vi "Example Bundler 2.vi"() -> ()   [LabVIEW 2014]
panel:
  out "ClusterIndicatorMy":cluster{string, i32, string[]}
  out "Error Out":errorcluster
  in  "Error In":errorcluster
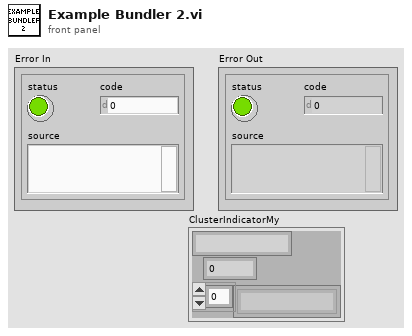
[diagram p1: front panel]
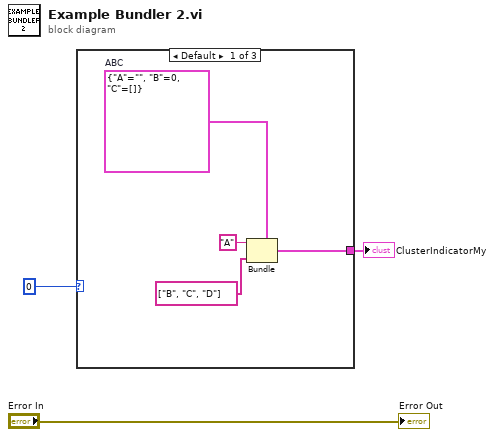
[diagram p0: block diagram]
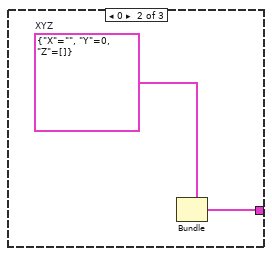
[diagram p2: hidden frame]
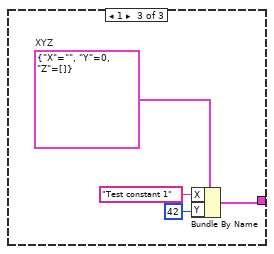
[diagram p3: hidden frame]
diagram:
  n1 = case shown="Default" 0 {
    tunnel: [w4 w8 w10] -> w1
    frame Default {
      w7 = cluster{"A":string, "B":i32, "C":string[]} {"A"="", "B"=0, "C"=[]}  # ABC
      n2 = Bundle(cluster=w7, "A"="A", "C"=string[] ["B", "C", "D"]) -> (w4:cluster{"A":string, "B":i32, "C":string[]})  [unwired: 1 in]
    }
    frame 0 {
      w9 = cluster{"X":string, "Y":i32, "Z":string[]} {"X"="", "Y"=0, "Z"=[]}  # XYZ
      n3 = Bundle(cluster=w9) -> (w8:cluster{"X":string, "Y":i32, "Z":string[]})  [unwired: 3 in]
    }
    frame 1 {
      w13 = cluster{"X":string, "Y":i32, "Z":string[]} {"X"="", "Y"=0, "Z"=[]}  # XYZ
      n4 = Bundle By Name(cluster=w13, "X"="Test constant 1", "Y"=42) -> (w10:cluster{"X":string, "Y":i32, "Z":string[]})
    }
  }
  "ClusterIndicatorMy" <- w1
  "Error Out" <- "Error In"
